vi "NavX Reset.vi"   [LabVIEW 2018]
uses:
  Robot Global Data.vi
types:
  T1 = cluster{"Yaw":dbl, "Roll":dbl, "Pitch":dbl, "Heading":dbl, "Fused Heading":dbl}
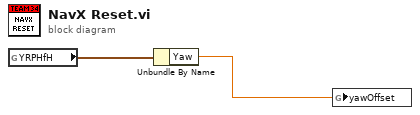
[diagram p0: block diagram]
diagram:
  n1 = global read "Robot Global Data.vi" "YRPHfH"() -> (w2:T1)
  n2 = Unbundle By Name(w2) -> ("Yaw"=w1:dbl)
  n3 = global write "Robot Global Data.vi" "yawOffset"(w1) -> ()
